vi "Main.vi"   [LabVIEW 2021]
uses:
  Child/Child.lvclass
  Parent/Parent.lvclass
  C:/PPLs/Decorating-Template-Method-with-Interfaces/Interface Inheritance and Interface Composition/Override and Call Interface/Override and Call Interface.lvclass
  Child/Child.lvclass/Child.ctl
  Child/Write Override and Call Interface.vi
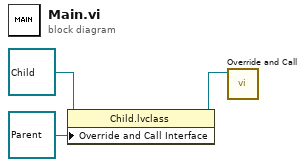
[diagram p0: block diagram]
diagram:
  n1 = property class="Child.lvclass"(reference=refnum<class "Child.lvclass"> refnum ("Child.lvclass"), "Override and Call Interface"=refnum<class "Parent.lvclass"> refnum ("Parent.lvclass")) -> (reference out=w2:refnum<class "Child.lvclass">)  [unwired: 1 in, 1 out]
  n2 = call-dynamic "Override and Call.vi"("Child in"=w2) -> ()  [unwired: 9 in, 2 out]
